vi "Position Open Mission Listbox.vi"(8 "error in (no error)":errorcluster, 11 "LstBox Refnum":refnum<vi>) -> (0 "error out":errorcluster)   [LabVIEW 2014]
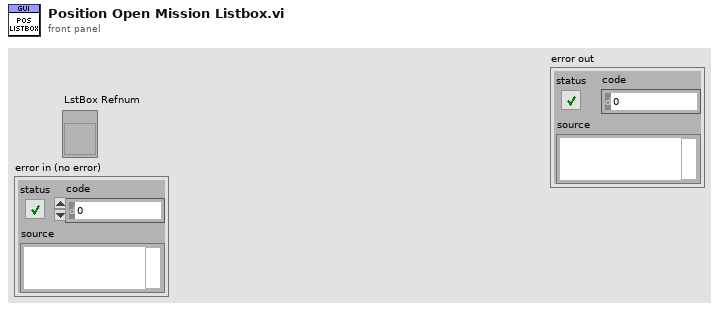
[diagram p1: front panel]
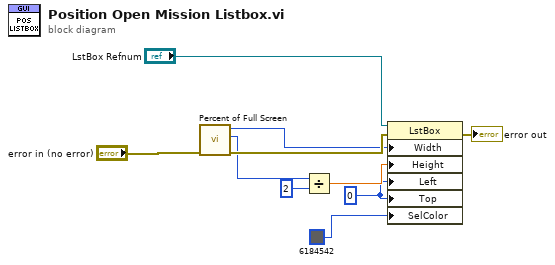
[diagram p0: block diagram]
diagram:
  w3 = 0 ("Position:Left")
  n1 = call "Percent of Full Screen.vi"("error in (no error)"="error in (no error)") -> ("error out"=w8:errorcluster, "Bottom"=w6:i16, "Right"=w7:i16)  [unwired: 8 in]
  n2 = Divide(x=w6, y=i16 2) -> (x/y=w4:dbl)
  n3 = property class="LstBox"(reference="LstBox Refnum", error in=w8, "Width"=w7, "Height"=w4, "Left"=w3, "Top"=w3, "SelColor"=u32 6184542) -> (error out=→"error out":errorcluster)  [unwired: 1 out]
